vi "Write Data.vi"(8 "error in (no error)":errorcluster, 9 "data_high":i32, 10 "data_low":i32, 11 "index":i32) -> (0 "error out":errorcluster, 3 "index_out":i32)   [LabVIEW 2013, in "FEMTO_LUCI-10.lvlib"]
doc: "This function writes data to the selected device.\nLow Byte - Pin 10-17\nHigh Byte - Pin 18-25"
uses:
  FEMTO_LUCI-10.lvlib
  LUCI_10.dll
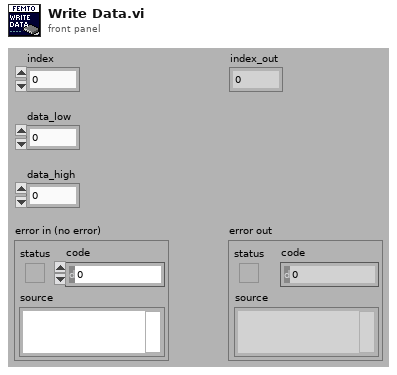
[diagram p1: front panel]
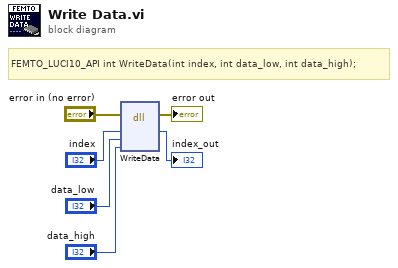
[diagram p0: block diagram]
diagram:
  # "FEMTO_LUCI10_API int WriteData(int index, int data_low, int data_high);"
  n1 = dll-call lib="C:/user/patrick/ppms_daq_femto/driver/LUCI_10.*" fn="WriteData"(error in="error in (no error)", "index"="index", "data_low"="data_low", "data_high"="data_high") -> (error out=→"error out":errorcluster, "index"=→"index_out":i32)  [unwired: 4 in, 2 out]
